vi "optomechanisc_AM2M.vi"() -> ()   [LabVIEW 2018]
panel:
  in  "VIS shutter":bool
  in  "stop":bool
  in  "VIS/IR":bool
  in  "VIS brigh. step [deg]":dbl=10.0
  in  "IR brigh. step [deg]":dbl=10.0
  in  "FIX refr step [mm]":dbl=3.0
  in  "VIS refr step [mm]":dbl=5.0
  in  "IR refr step [mm]":dbl=5.0
  in  "IR shutter":bool
  in  "Adjust VIS brightness":bool
  in  "Adjust IR brightness":bool
  in  "Set FIXATION refraction":bool
  in  "Set VIS refraction":bool
  in  "Set IR refraction":bool
  in  "OK Button":bool
  in  "SM set power [W]":dbl=6e-07
  out "Test optotype":cluster{"sine wave":dbl[], "sine wave":dbl[]}(graph)={"sine wave"=[0.0, 0.002453383716370901, 0.0049008570164780305, 0.007336523722768088, 0.009754516100806413, 0.012149008995163194, 0.014514233862723118, 0.016844492669611, 0.019134171618254488, 0.021377754671514104, 0.02356983684129988, 0.025705137209661083, 0.02777851165098011, 0.029784965224621665, 0.03171966420818227, 0.03357794774235092, 0.035355339059327376, 0.03704755626774796, 0.038650522668136844, 0.04016037657403225, 0.04157348061512726, 0.04288643050001361, 0.04409606321741775, 0.045199464656172174, 0.046193976625564334, 0.047077203259151046, 0.047847016786610436, 0.04850156265972721, 0.04903926402016152, 0.04945882549823906, 0.04975923633360984, 0.04993977281025863, 0.049999999999999996, 0.04993977281025863, 0.04975923633360984, 0.04945882549823906, 0.04903926402016152, 0.04850156265972721, 0.047847016786610436, 0.047077203259151046, 0.04619397662556433, 0.045199464656172174, 0.04409606321741774, 0.04288643050001361, 0.04157348061512725, 0.04016037657403225, 0.03865052266813684, 0.03704755626774796, 0.03535533905932737, 0.03357794774235092, 0.03171966420818227, 0.029784965224621665, 0.02777851165098011, 0.025705137209661083, 0.02356983684129988, 0.0213777546715141, 0.019134171618254488, 0.016844492669610998, 0.014514233862723118, 0.012149008995163189, 0.009754516100806413, 0.007336523722768081, 0.00490085701647803, 0.002453383716370893, 0.0, -0.0024533837163709096, -0.00490085701647803, -0.007336523722768097, -0.009754516100806413, -0.012149008995163205, -0.014514233862723117, -0.016844492669611015, -0.019134171618254488, -0.021377754671514117, -0.02356983684129988, -0.0257051372096611, -0.02777851165098011, -0.029784965224621682, -0.03171966420818227, -0.033577947742350935, -0.03535533905932737, -0.03704755626774797, -0.03865052266813684, -0.040160376574032264, -0.04157348061512725, -0.042886430500013624, -0.04409606321741774, -0.04519946465617219, -0.04619397662556433, -0.04707720325915106, -0.047847016786610436, -0.04850156265972722, -0.04903926402016152, -0.04945882549823907, -0.04975923633360984, -0.049939772810258645, -0.049999999999999996, -0.049939772810258645, -0.04975923633360984, -0.04945882549823907, -0.04903926402016152, -0.04850156265972722, -0.047847016786610436, -0.04707720325915106, -0.04619397662556433, -0.04519946465617219, -0.04409606321741774, -0.042886430500013624, -0.04157348061512725, -0.040160376574032264, -0.03865052266813684, -0.03704755626774797, -0.03535533905932737, -0.033577947742350935, -0.03171966420818227, -0.02978496522462168, -0.02777851165098011, -0.025705137209661093, -0.02356983684129988, -0.021377754671514107, -0.019134171618254488, -0.016844492669611, -0.014514233862723118, -0.012149008995163189, -0.009754516100806413, -0.007336523722768078, -0.00490085701647803, -0.002453383716370887], "sine wave"=[0.05, 0.049939772810258624, 0.049759236333609846, 0.04945882549823905, 0.049039264020161524, 0.0485015626597272, 0.04784701678661044, 0.04707720325915104, 0.046193976625564334, 0.04519946465617217, 0.04409606321741775, 0.0428864305000136, 0.04157348061512726, 0.04016037657403224, 0.038650522668136844, 0.03704755626774795, 0.035355339059327376, 0.033577947742350914, 0.03171966420818227, 0.02978496522462166, 0.02777851165098011, 0.025705137209661083, 0.02356983684129988, 0.0213777546715141, 0.019134171618254488, 0.016844492669610998, 0.014514233862723117, 0.01214900899516319, 0.00975451610080641, 0.007336523722768084, 0.004900857016478025, 0.0024533837163708975, -6.071532165918825e-18, -0.0024533837163709035, -0.0049008570164780375, -0.00733652372276809, -0.009754516100806422, -0.012149008995163198, -0.014514233862723127, -0.016844492669611005, -0.019134171618254498, -0.021377754671514107, -0.023569836841299895, -0.025705137209661087, -0.027778511650980123, -0.029784965224621665, -0.031719664208182285, -0.033577947742350914, -0.03535533905932739, -0.037047556267747944, -0.03865052266813686, -0.040160376574032236, -0.04157348061512727, -0.042886430500013596, -0.04409606321741776, -0.04519946465617216, -0.04619397662556435, -0.04707720325915103, -0.04784701678661045, -0.048501562659727195, -0.04903926402016153, -0.049458825498239045, -0.04975923633360985, -0.04993977281025862, -0.05, -0.04993977281025862, -0.049759236333609846, -0.049458825498239045, -0.049039264020161524, -0.048501562659727195, -0.04784701678661044, -0.04707720325915103, -0.046193976625564334, -0.04519946465617216, -0.04409606321741775, -0.042886430500013596, -0.04157348061512726, -0.040160376574032236, -0.038650522668136844, -0.037047556267747944, -0.03535533905932737, -0.033577947742350914, -0.031719664208182265, -0.02978496522462166, -0.0277785116509801, -0.025705137209661083, -0.023569836841299867, -0.021377754671514104, -0.01913417161825447, -0.016844492669611, -0.0145142338627231, -0.012149008995163194, -0.009754516100806392, -0.007336523722768088, -0.004900857016478009, -0.002453383716370901, 2.168404344971009e-17, 0.0024533837163709, 0.004900857016478052, 0.007336523722768087, 0.009754516100806436, 0.012149008995163194, 0.01451423386272314, 0.016844492669611, 0.019134171618254512, 0.021377754671514104, 0.023569836841299905, 0.025705137209661083, 0.027778511650980133, 0.02978496522462166, 0.0317196642081823, 0.033577947742350914, 0.035355339059327404, 0.037047556267747944, 0.03865052266813687, 0.040160376574032236, 0.041573480615127285, 0.042886430500013596, 0.044096063217417776, 0.04519946465617216, 0.04619397662556436, 0.04707720325915103, 0.04784701678661046, 0.048501562659727195, 0.04903926402016154, 0.049458825498239045, 0.04975923633360986, 0.04993977281025862]}
  # "Optotype"
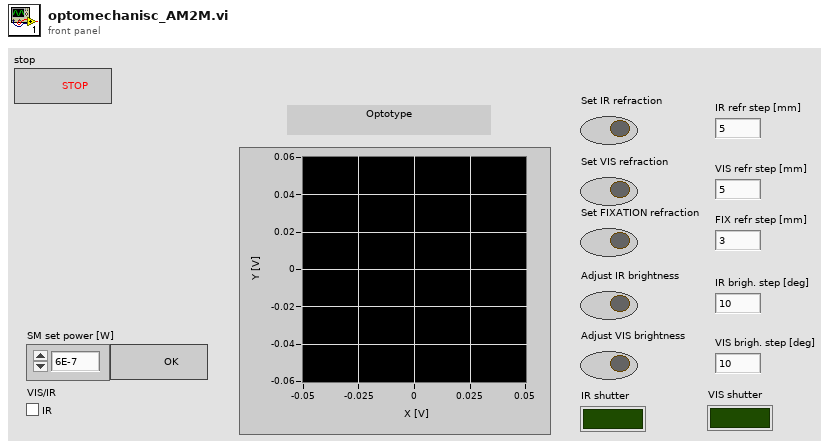
[diagram p1: front panel]
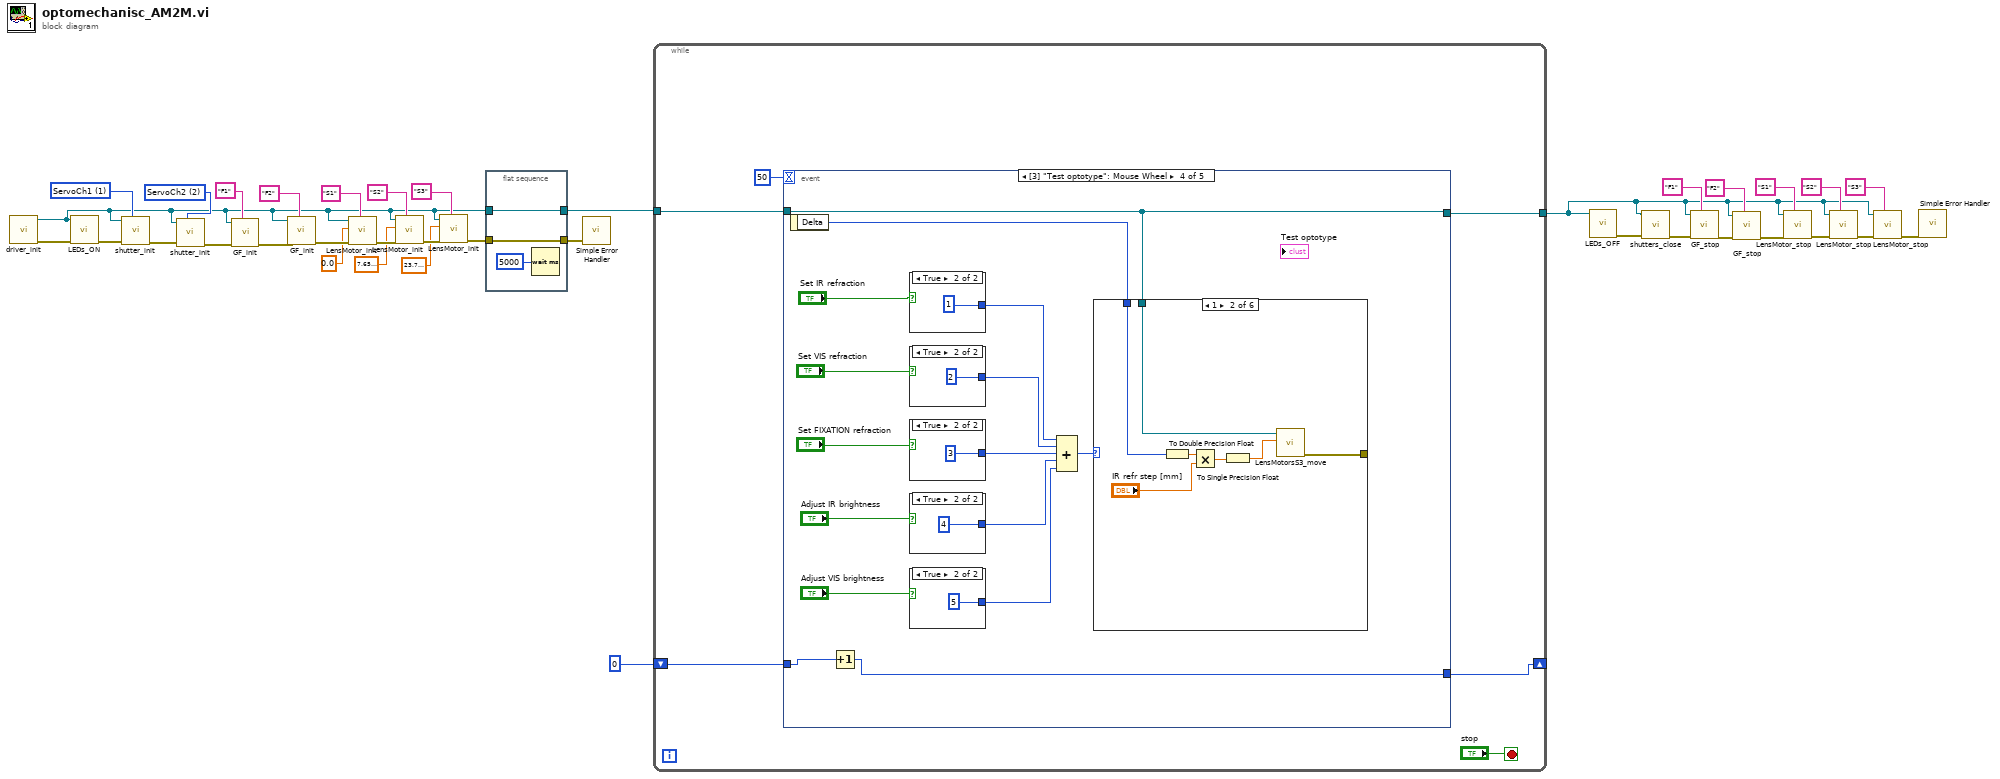
[diagram p0: block diagram]
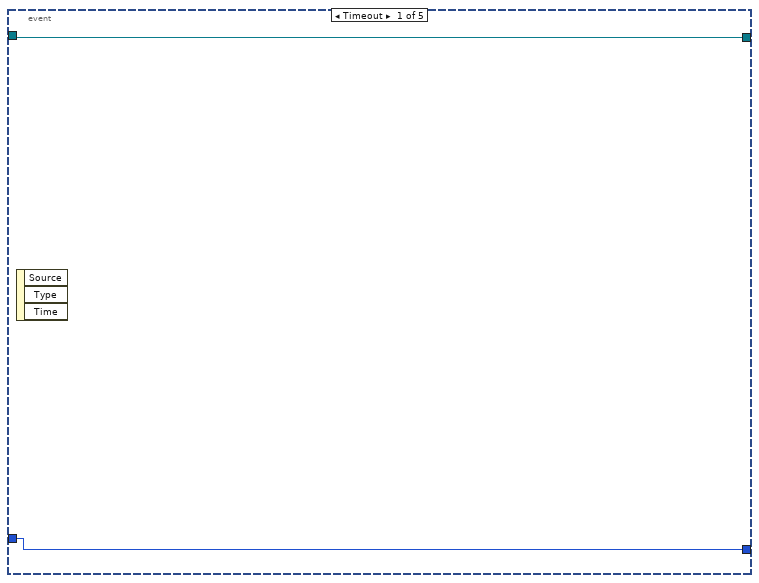
[diagram p2: hidden frame]
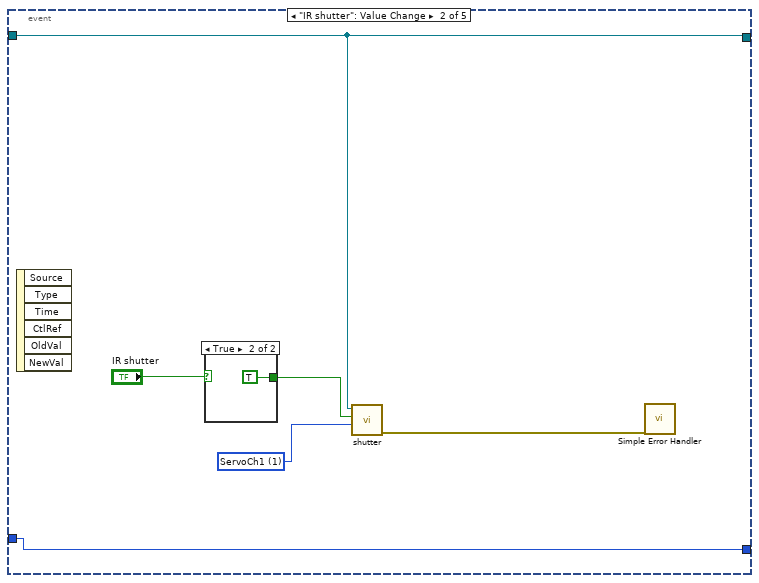
[diagram p3: hidden frame]
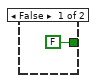
[diagram p4: hidden frame]
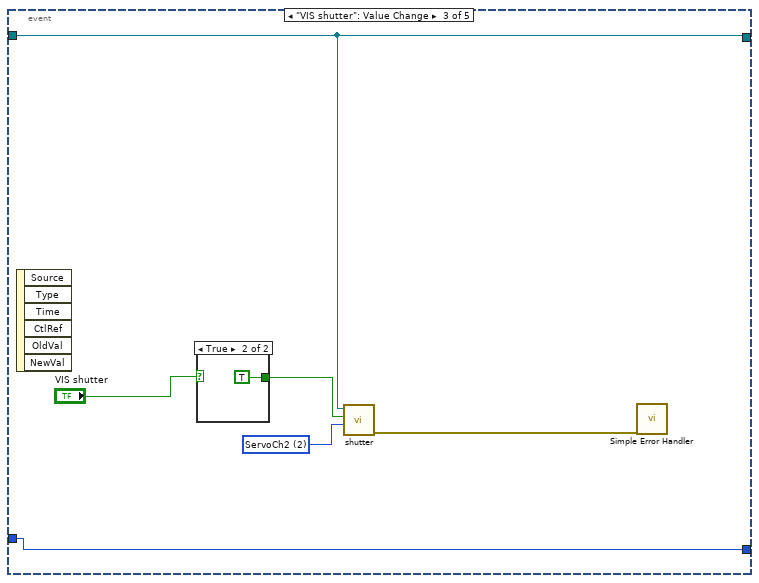
[diagram p5: hidden frame]
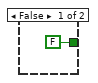
[diagram p6: hidden frame]
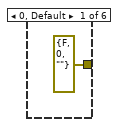
[diagram p7: hidden frame]
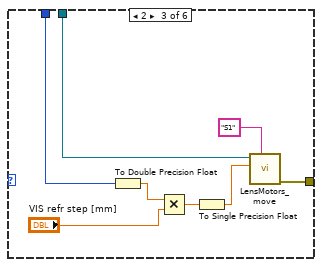
[diagram p8: hidden frame]
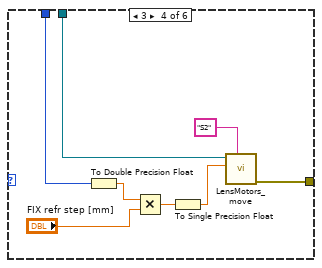
[diagram p9: hidden frame]
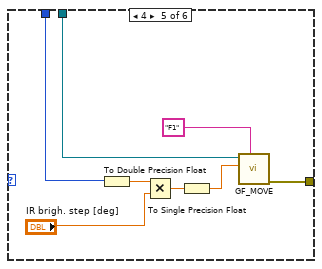
[diagram p10: hidden frame]
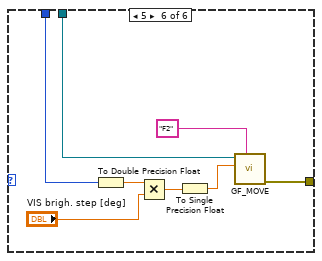
[diagram p11: hidden frame]
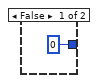
[diagram p12: hidden frame]
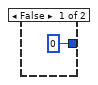
[diagram p13: hidden frame]
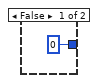
[diagram p14: hidden frame]
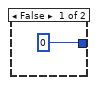
[diagram p15: hidden frame]
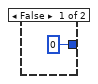
[diagram p16: hidden frame]
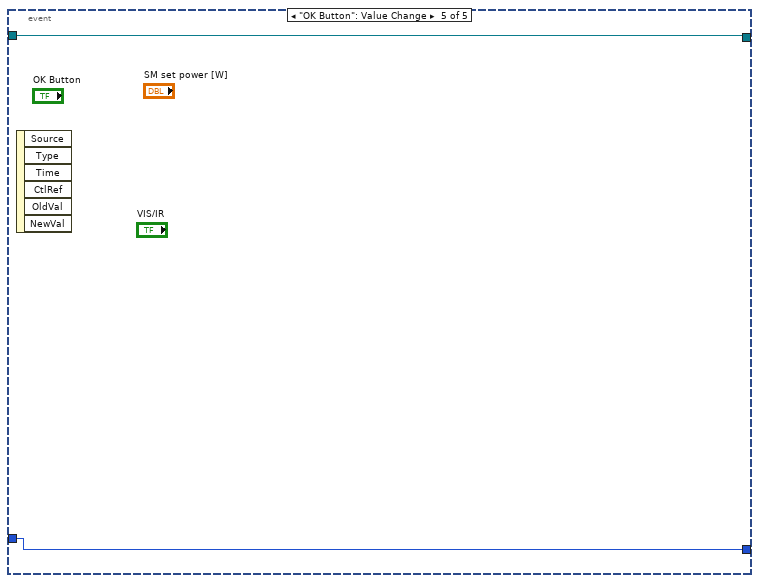
[diagram p17: hidden frame]
diagram:
  w27 = 2 items=["ServoUnspecified", "ServoCh1", "ServoCh2", "ServoBoth"] ("servo")
  w28 = 1 items=["ServoUnspecified", "ServoCh1", "ServoCh2", "ServoBoth"] ("servo")
  n1 = call "driver_init.vi"() -> ("error out"=w34:errorcluster, "new reference"=w12:refnum<k24>)  [unwired: 10 in]
  n2 = call "LEDs_ON.vi"("error in (no error)"=w34, "channel"=w12) -> ("error out"=w35:errorcluster)  [unwired: 9 in]
  n3 = call "shutter_init.vi"("servo"=w28, "error in (no error)"=w35, "channel"=w12) -> ("error out"=w29:errorcluster)  [unwired: 8 in]
  n4 = call "shutter_init.vi"("servo"=w27, "error in (no error)"=w29, "channel"=w12) -> ("error out"=w26:errorcluster)  [unwired: 8 in]
  n5 = call "GF_init.vi"("modIdTag"="F1", "error in (no error)"=w26, "channel"=w12) -> ("error out"=w25:errorcluster)  [unwired: 8 in]
  n6 = call "GF_init.vi"("modIdTag"="F2", "error in (no error)"=w25, "channel"=w12) -> ("error out"=w36:errorcluster)  [unwired: 8 in]
  n7 = call "LensMotor_init.vi"("modIdTag"="S1", "error in (no error)"=w36, "position"=sgl 0.0, "channel"=w12) -> ("error out"=w22:errorcluster)  [unwired: 7 in]
  n8 = call "LensMotor_init.vi"("modIdTag"="S2", "error in (no error)"=w22, "position"=sgl 7.65, "channel"=w12) -> ("error out"=w21:errorcluster)  [unwired: 7 in]
  n9 = call "LensMotor_init.vi"("modIdTag"="S3", "error in (no error)"=w21, "position"=sgl 23.7, "channel"=w12) -> ("error out"=w14:errorcluster)  [unwired: 7 in]
  n10 = flat-sequence {
    tunnel: w14 -> [w39]
    tunnel: [w39] -> w13
    tunnel: w12 -> [w38]
    tunnel: [w38] -> w11
    frame #0 {
      n11 = Wait (ms)(milliseconds to wait=u32 5000) -> ()  [unwired: 1 out]
    }
  }
  n12 = call <vilib>:"Simple Error Handler.vi"("error in (no error)"=w13) -> ()  [unwired: 4 in, 5 out]
  n13 = while {
    tunnel: w11 -> [w43]
    tunnel: [w42] -> w2
    shift-right: [w40] -> _
    shift-left: 0 -> [w41]
    stop <- "stop" stop-if-true
    n14 = event shown="[3] \"Test optotype\": Mouse Wheel" {
      selector: _ -> [_ _ _ _ _]
      dyn-events: _ -> [_ _ _ _ _]
      timeout: 50 -> [_ _ _ _ _]
      tunnel: w43 -> [w47 w49 w58 w66 w130]
      tunnel: [w47 w49 w58 w66 w130] -> w42
      tunnel: w41 -> [w46 w48 w56 w65 w129]
      tunnel: [w46 w48 w56 w64 w129] -> w40
      event Timeout {
        n15 = event-data() -> ()  [unwired: 1 in, 3 out]
      }
      event "IR shutter": Value Change {
        w52 = 1 items=["ServoUnspecified", "ServoCh1", "ServoCh2", "ServoBoth"] ("servo")
        n16 = event-data() -> ()  [unwired: 1 in, 6 out]
        n17 = case shown="True" "IR shutter" {
          tunnel: [FALSE ("Status") TRUE ("Status")] -> w53
          frame False {
          }
          frame True {
          }
        }
        n18 = call "shutter.vi"("servo"=w52, "Status"=w53, "channel"=w49) -> ("error out"=w51:errorcluster)  [unwired: 8 in]
        n19 = call <vilib>:"Simple Error Handler.vi"("error in (no error)"=w51) -> ()  [unwired: 4 in, 5 out]
      }
      event "VIS shutter": Value Change {
        w59 = 2 items=["ServoUnspecified", "ServoCh1", "ServoCh2", "ServoBoth"] ("servo")
        n20 = event-data() -> ()  [unwired: 1 in, 6 out]
        n21 = case shown="True" "VIS shutter" {
          tunnel: [FALSE ("Status") TRUE ("Status")] -> w60
          frame False {
          }
          frame True {
          }
        }
        n22 = call "shutter.vi"("servo"=w59, "Status"=w60, "channel"=w58) -> ("error out"=w61:errorcluster)  [unwired: 8 in]
        n23 = call <vilib>:"Simple Error Handler.vi"("error in (no error)"=w61) -> ()  [unwired: 4 in, 5 out]
      }
      event "Test optotype": Mouse Wheel {
        n24 = event-data() -> ("Delta"=w72:i32)  [unwired: 1 in]
        n25 = Increment(x=w65) -> (x+1=w64:i32)
        n26 = case shown="True" "Set IR refraction" {
          tunnel: [0 1] -> w77
          frame False {
          }
          frame True {
          }
        }
        n27 = case shown="True" "Set VIS refraction" {
          tunnel: [0 2] -> w76
          frame False {
          }
          frame True {
          }
        }
        n28 = case shown="True" "Set FIXATION refraction" {
          tunnel: [0 3] -> w75
          frame False {
          }
          frame True {
          }
        }
        n29 = case shown="True" "Adjust IR brightness" {
          tunnel: [0 4] -> w73
          frame False {
          }
          frame True {
          }
        }
        n30 = case shown="True" "Adjust VIS brightness" {
          tunnel: [0 5] -> w74
          frame False {
          }
          frame True {
          }
        }
        n31 = Compound Arithmetic op=ADD(w77, w76, w75, w73, w74) -> (w78:i32)
        n32 = case shown="1" w78 {
          tunnel: [errorcluster {"status"=FALSE, "code"=0, "source"=""} ("error out") w86 w93 w98 w110 w116] -> _
          tunnel: w66 -> [_ w82 w89 w97 w105 w113]
          tunnel: w72 -> [_ w81 w88 w96 w103 w112]
          frame 0, Default {
          }
          frame 1 {
            n33 = To Double Precision Float(number=w81) -> (double precision float=w83:dbl)
            n34 = Multiply(x=w83, y="IR refr step [mm]") -> (x*y=w85:dbl)
            n35 = To Single Precision Float(number=w85) -> (single precision float=w84:sgl)
            n36 = call "LensMotorsS3_move.vi"("delta"=w84, "channel"=w82) -> ("error out"=w86:errorcluster)  [unwired: 9 in]
          }
          frame 2 {
            n37 = To Double Precision Float(number=w88) -> (double precision float=w92:dbl)
            n38 = Multiply(x=w92, y="VIS refr step [mm]") -> (x*y=w91:dbl)
            n39 = To Single Precision Float(number=w91) -> (single precision float=w90:sgl)
            n40 = call "LensMotors_move.vi"("modIdTag"="S1", "delta"=w90, "channel"=w89) -> ("error out"=w93:errorcluster)  [unwired: 8 in]
          }
          frame 3 {
            n41 = To Double Precision Float(number=w96) -> (double precision float=w100:dbl)
            n42 = Multiply(x=w100, y="FIX refr step [mm]") -> (x*y=w101:dbl)
            n43 = To Single Precision Float(number=w101) -> (single precision float=w102:sgl)
            n44 = call "LensMotors_move.vi"("modIdTag"="S2", "delta"=w102, "channel"=w97) -> ("error out"=w98:errorcluster)  [unwired: 8 in]
          }
          frame 4 {
            n45 = To Double Precision Float(number=w103) -> (double precision float=w108:dbl)
            n46 = Multiply(x=w108, y="IR brigh. step [deg]") -> (x*y=w107:dbl)
            n47 = To Single Precision Float(number=w107) -> (single precision float=w106:sgl)
            n48 = call "GF_MOVE.vi"("modIdTag"="F1", "delta"=w106, "channel"=w105) -> ("error out"=w110:errorcluster)  [unwired: 8 in]
          }
          frame 5 {
            n49 = To Double Precision Float(number=w112) -> (double precision float=w118:dbl)
            n50 = Multiply(x=w118, y="VIS brigh. step [deg]") -> (x*y=w115:dbl)
            n51 = To Single Precision Float(number=w115) -> (single precision float=w114:sgl)
            n52 = call "GF_MOVE.vi"("modIdTag"="F2", "delta"=w114, "channel"=w113) -> ("error out"=w116:errorcluster)  [unwired: 8 in]
          }
        }
      }
      event "OK Button": Value Change {
        n53 = event-data() -> ()  [unwired: 1 in, 6 out]
      }
    }
  }
  n54 = call "LEDs_OFF.vi"("channel"=w2) -> ("error out"=w33:errorcluster)  [unwired: 10 in]
  n55 = call "shutters_close.vi"("error in (no error)"=w33, "channel"=w2) -> ("error out"=w32:errorcluster)  [unwired: 9 in]
  n56 = call "GF_stop.vi"("modIdTag"="F1", "error in (no error)"=w32, "channel"=w2) -> ("error out"=w10:errorcluster)  [unwired: 8 in]
  n57 = call "GF_stop.vi"("modIdTag"="F2", "error in (no error)"=w10, "channel"=w2) -> ("error out"=w7:errorcluster)  [unwired: 8 in]
  n58 = call "LensMotor_stop.vi"("modIdTag"="S1", "error in (no error)"=w7, "channel"=w2) -> ("error out"=w6:errorcluster)  [unwired: 8 in]
  n59 = call "LensMotor_stop.vi"("modIdTag"="S2", "error in (no error)"=w6, "channel"=w2) -> ("error out"=w5:errorcluster)  [unwired: 8 in]
  n60 = call "LensMotor_stop.vi"("modIdTag"="S3", "error in (no error)"=w5, "channel"=w2) -> ("error out"=w31:errorcluster)  [unwired: 8 in]
  n61 = call <vilib>:"Simple Error Handler.vi"("error in (no error)"=w31) -> ()  [unwired: 4 in, 5 out]
